vi "FPGA Main.vi"() -> ()   [LabVIEW 2016]
uses:
  <vilib>/Platform/TimedLoop/XDataNode/timing_clust.ctl
  <vilib>/Platform/TimedLoop/XDataNode/nitl_modes.ctl
  <vilib>/Platform/TimedLoop/XDataNode/wakeup.ctl
  <vilib>/rvi/Emulation/niFpgaSctlEmulationGetInTimedLoop.vi
  <vilib>/rvi/Emulation/niFpgaEmulationReportErrorSimple.vi
  <vilib>/rvi/Emulation/niFpgaGetClockAttributes.vi
  <vilib>/rvi/Emulation/niFpgaCriticalErrorInLSC.vi
  <vilib>/rvi/interface/RandomDataEmulation/niFpgaRandomDataHandleErrors.vi
  <vilib>/Platform/TimedLoop/XDataNode/XDataNode.xnode
  <vilib>/rvi/DataTransferAndStorage/Container/XNode/niFpgaContainer.xnode
  <vilib>/rvi/interface/RandomDataEmulation/nirviRandomDataFpgaReadWriteTemplate.vi
  <vilib>/Platform/TimedLoop/XDataNode/XDNodeRunTimeDep.lvlib
panel:
  in  "Number of Pixe":u32=256
  in  "Upper Threhold (counts)":u32
  in  "Dwell Time (#80MHz SCTLs)":u32=8000
  in  "T3":u32=1000
  in  "T2":u32=1000
  in  "T1":u32=1000
  in  "T0":u32=1000
  in  "t3":u32=1000
  in  "t2":u32=1000
  in  "t1":u32=1000
  in  "t0":u32=1000
  in  "V3":u16=1000
  in  "V2":i16=1000
  in  "V1":i16=232
  in  "V0":u16=1000
  out "Overflow1":bool
  out "Overflow2":bool
  in  "Dymin On?":bool
  in  "stop 4":bool
  in  "stop 3":bool
  in  "stop 2":bool
  in  "stop 1":bool
  # "Reminder:These \"Volts\" are actually in bits.  Use  the RT_Main vi to run this code by inputting actual Volts.  Floats aren't possible in an FPGA program."
  # "Step before step with tn=0 is the last Dymin Step, threshold is ignored on last step, just count APD counts in selected time"
  # "AOM Voltage (bits)"
  # "Times (#80MHz periods)"
  # "Threshold (counts)"
  # "16=200ns\n32=400ns"
  # "nominal 12 bit ADC volts"
  # ".1=82\n.2=164\n.3=246"
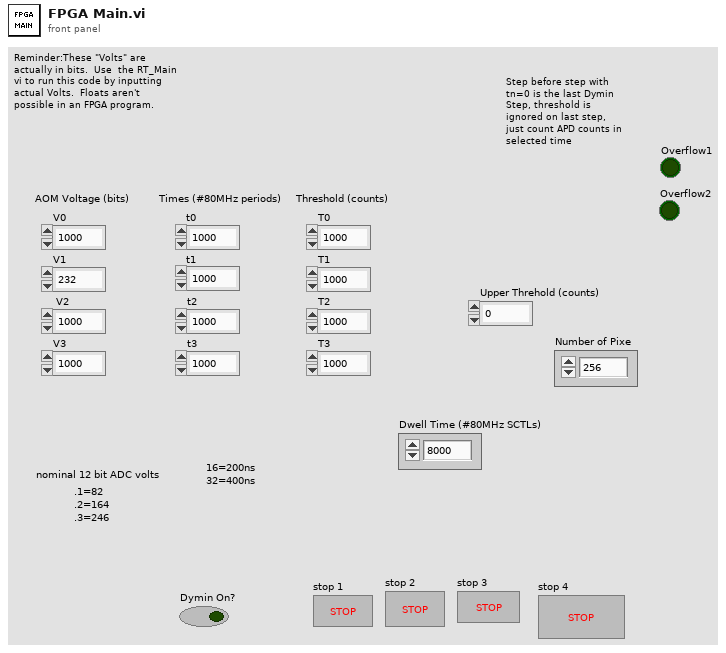
[diagram p1: front panel]
types:
  T1 = typedef "XDNodeRunTimeDep.lvlib/timing_clust.ctl" = cluster{"Expected End [f-1]":u64, "Actual End [f-1]":u64, "Finished Late? [f-1]":bool, "Expected End [i-1]":u64, "Actual End [i-1]":u64, "Finished Late? [i-1]":bool, "Expected Start [i]":u64, "Actual Start [i]":u64, "Expected Start [f]":u64, "Actual Start [f]":u64, "Source Name":string, "Structure Name":string, "Period":i64, "Deadline":i64, "Offset":i64, "Start":i64, "Priority":i32, "Timeout":i32, "Mode":T2, "Wakeup Reason":T3, "Error":errorcluster, "Source Type":string, "Secondary Source Type":string, "Global End Time":u64, "Global Start Time":u64, "Frame Duration":u64, "Iteration Duration":u64, "Assigned CPU":i32, "I/O Scan Engine Mode":u32}
  T2 = typedef "XDNodeRunTimeDep.lvlib/nitl_modes.ctl" = enum32{"No Change", "Process missed periods, maintain original phase", "Discard missed periods, maintain original phase", "Process missed periods, ignore original phase", "Discard missed periods, ignore original phase"}
  T3 = typedef "XDNodeRunTimeDep.lvlib/wakeup.ctl" = enum32{"Normal", "Aborted", "Asynchronous wakeup", "Timing source error", "Timed loop error", "Timeout"}
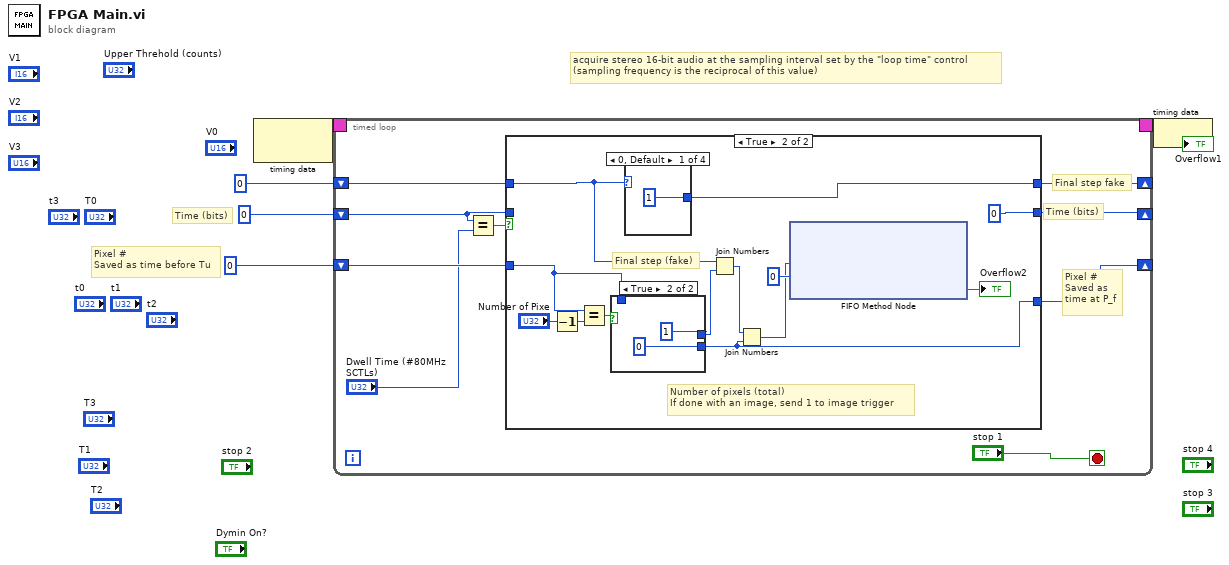
[diagram p0: block diagram]
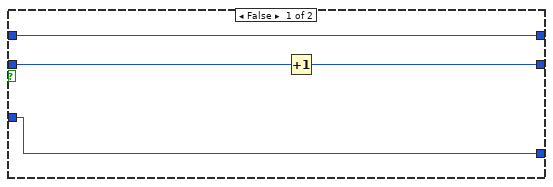
[diagram p2: hidden frame]
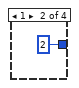
[diagram p3: hidden frame]
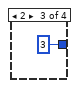
[diagram p4: hidden frame]
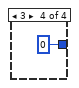
[diagram p5: hidden frame]
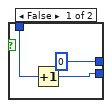
[diagram p6: hidden frame]
diagram:
  # "Pixel #\nSaved as time before Tu"
  # "Time (bits)"
  # "acquire stereo 16-bit audio at the sampling interval set by the \"loop time\" control\n(sampling frequency is the reciprocal of this value)"
  n1 = node-c288() -> (w5:T1)  [unwired: 1 in]
  n2 = timed-loop {
    timing: w5 -> [_]
    timing-out: [_] -> w4
    shift-right: [w12] -> _
    shift-left: u32 0 -> [w13]
    shift-right: [w9] -> _
    shift-left: u16 0 -> [w10]
    shift-right: [w7] -> _
    shift-left: u32 0 -> [w11]
    stop <- "stop 1" stop-if-true
    # "Pixel #\nSaved as\ntime at P_f"
    # "Final step fake"
    # "Time (bits)"
    n3 = Equal?(x=w13, y="Dwell Time (#80MHz SCTLs)") -> (x = y?=w14:bool)
    n4 = case shown="True" w14 {
      tunnel: w13 -> [w18 _]
      tunnel: [w17 u32 0] -> w12
      tunnel: w11 -> [w15 w22]
      tunnel: w10 -> [w16 w27]
      tunnel: [w16 w28] -> w9
      tunnel: [w15 w21] -> w7
      frame False {
        n5 = Increment(x=w18) -> (x+1=w17:u32)
      }
      frame True {
        # "Final step (fake)"
        # "Number of pixels (total)\nIf done with an image, send 1 to image trigger"
        n6 = Decrement(x="Number of Pixe") -> (x-1=w19:u32)
        n7 = Equal?(x=w22, y=w19) -> (x = y?=w29:bool)
        n8 = case shown="True" w29 {
          tunnel: [u16 0 u16 1] -> w26
          tunnel: w22 -> [w37 _]
          tunnel: [w36 u32 0] -> w21
          frame False {
            n9 = Increment(x=w37) -> (x+1=w36:u32)
          }
          frame True {
          }
        }
        n10 = case shown="0, Default" w27 {
          tunnel: [u16 1 u16 2 u16 3 u16 0] -> w28
          frame 0, Default {
          }
          frame 1 {
          }
          frame 2 {
          }
          frame 3 {
          }
        }
        n11 = Join Numbers(hi=w27, lo=w26) -> ((hi.lo)=w25:u32)
        n12 = Join Numbers(hi=w25, lo=w21) -> ((hi.lo)=w24:u64)
        n13 = xnode "FIFO Method Node"("Element"=w24, "Timeout"=0) -> ("Timed Out?"=→"Overflow2":bool)  [unwired: 1 in, 1 out]
      }
    }
  }
  n14 = node-c288(w4) -> ()
